vi "Actor Core.vi"(8 "error in":errorcluster, 11 "Nested in":refnum<class "Chef Actor.lvclass">) -> (0 "error out":errorcluster, 3 "Actor out":refnum<class "Actor.lvclass">)   [LabVIEW 2024, in "Chef Actor.lvlib" / "Chef Actor.lvclass"]
doc: "(<B>Filename</B>: Actor Framework.lvlib:Actor.lvclass:Actor Core.vi)\n\nReceives messages to the actor, reacts to them, and initiates any error handling that may shut the actor down.\n\nDescendant classes may override this VI to append parallel tasks for the actor to complete while it handles messages. Overrides use the Call Parent Method node."
uses:
  Chef Actor.lvclass
  C:/Program Files/National Instruments/LabVIEW 2024/vi.lib/ActorFramework/Actor/Actor.lvclass
  <vilib>/ActorFramework/Actor/Actor.lvclass
  Support/Step.ctl
  Timer/Timer/Timer.lvclass
  Cooker Actor/Cooker Actor.lvclass
  <vilib>/ActorFramework/Actor/Actor.lvclass/Actor.ctl
  <vilib>/ActorFramework/Message Enqueuer/Message Enqueuer.lvclass/Message Enqueuer.ctl
  Chef Actor.lvclass/Chef Actor.ctl
  <vilib>/ActorFramework/Message Enqueuer/Message Priority.ctl
  Chef Actor Messages/Start Cooker Msg/Start Cooker Msg.lvclass/Start Cooker Msg.ctl
  Chef Actor Messages/Start Timer Msg/Start Timer Msg.lvclass/Start Timer Msg.ctl
  <vilib>/ActorFramework/Message Enqueuer/Init from Existing Queue.vi
  <vilib>/ActorFramework/Message Enqueuer/Enqueue.vi
  Chef Actor Messages/Stop Timer Msg/Stop Timer Msg.lvclass
  C:/Program Files/National Instruments/LabVIEW 2024/vi.lib/ActorFramework/Message/Message.lvclass
  <vilib>/ActorFramework/Stop Msg/Stop Msg.lvclass
  Chef Actor Messages/Start Cooker Msg/Start Cooker Msg.lvclass
  Chef Actor Messages/Start Timer Msg/Start Timer Msg.lvclass
  <vilib>/ActorFramework/Message Priority Queue/Priority Enqueue.vi
  <vilib>/ActorFramework/Message Enqueuer/Message Enqueuer.lvclass
panel:
  out "Real Elapsed Time":u32
  out "Start Time":u32
  in  "StepsTable":string[][](table)
  out "StepsControl":T1[](array[typedef]) {"Duration" min=0.0 max=100.0 format="%.2f"; "Fire" min=0.0 max=100.0 format="%.2f %"}
  in  "Exit Button":bool
  out "Go Next Step":bool
  out "Current Index":i32
  out "Elapsed TÝme - Signal":bool
  in  "Start Button":bool
  out "Time Elapsed":dbl min=0.0 max=100.0 format="%.4f"
  # "STEPS"
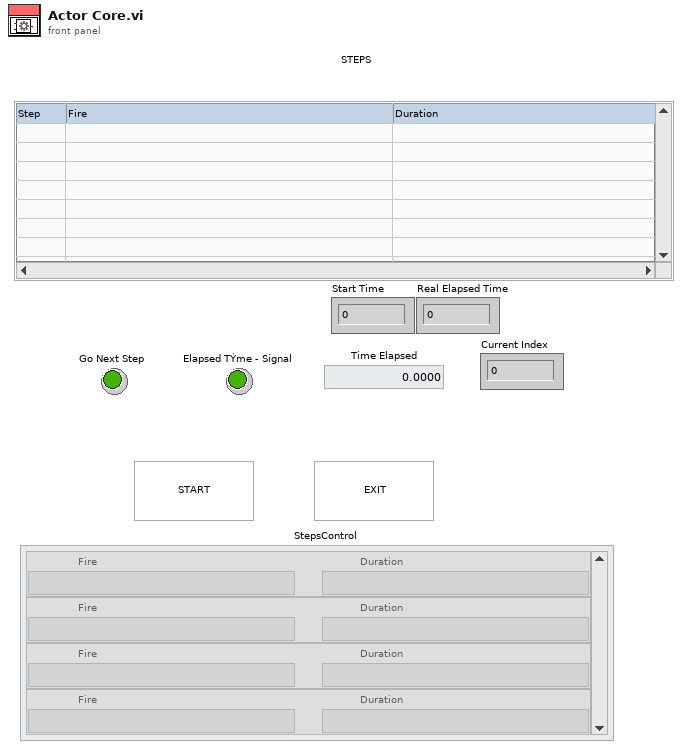
[diagram p1: front panel]
types:
  T1 = typedef "Step.ctl" = cluster{"Fire":dbl, "Duration":dbl}
  T2 = cluster{"Stop":refnum<user-event>, "Update Time Elapsed":refnum<user-event>, "Go Next Step":refnum<user-event>}
  T3 = typedef "Actor Framework.lvlib/Message Enqueuer.lvclass/Message Priority.ctl" = enum16{"Low", "Normal", "High"}
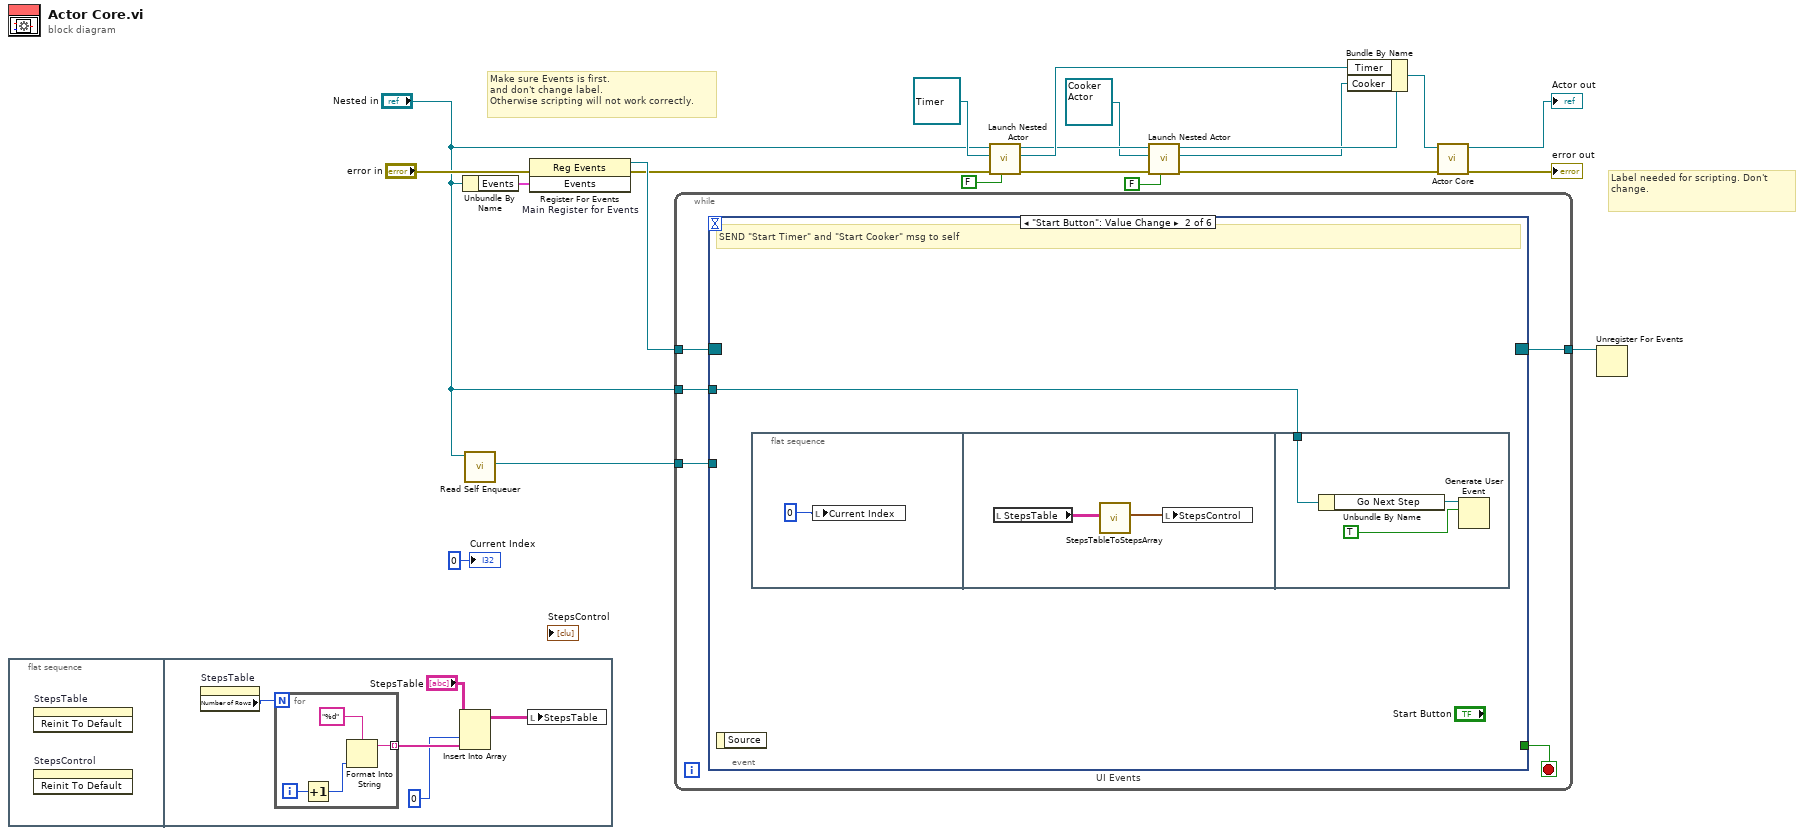
[diagram p0: block diagram]
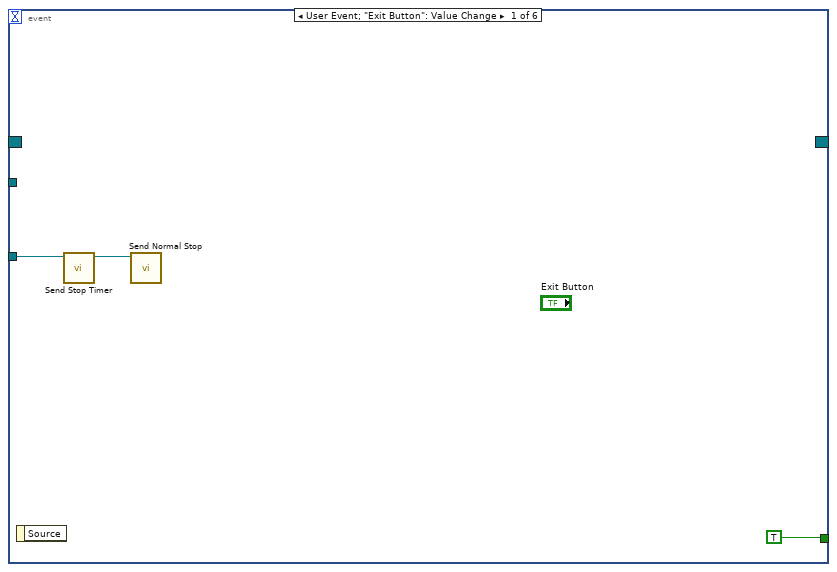
[diagram p2: hidden frame]
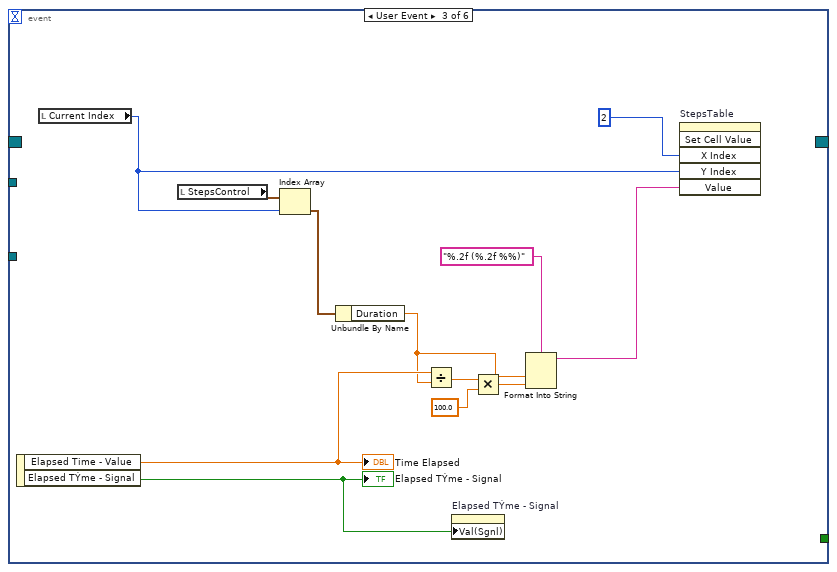
[diagram p3: hidden frame]
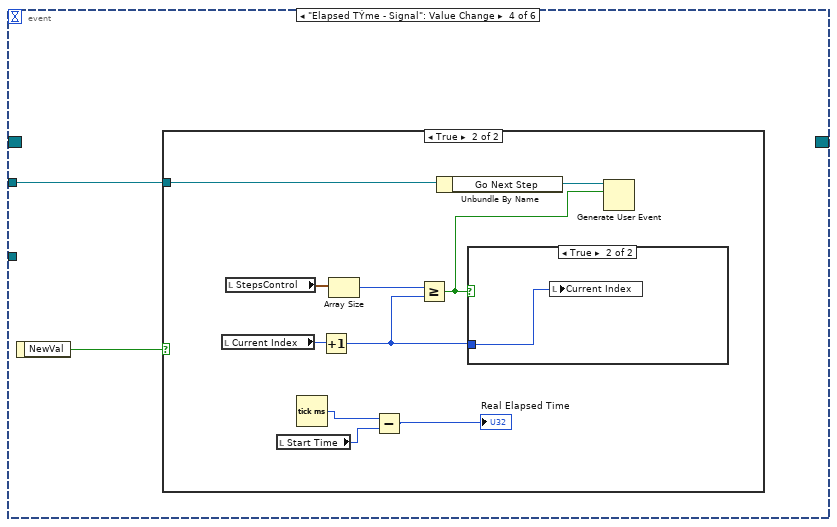
[diagram p4: hidden frame]
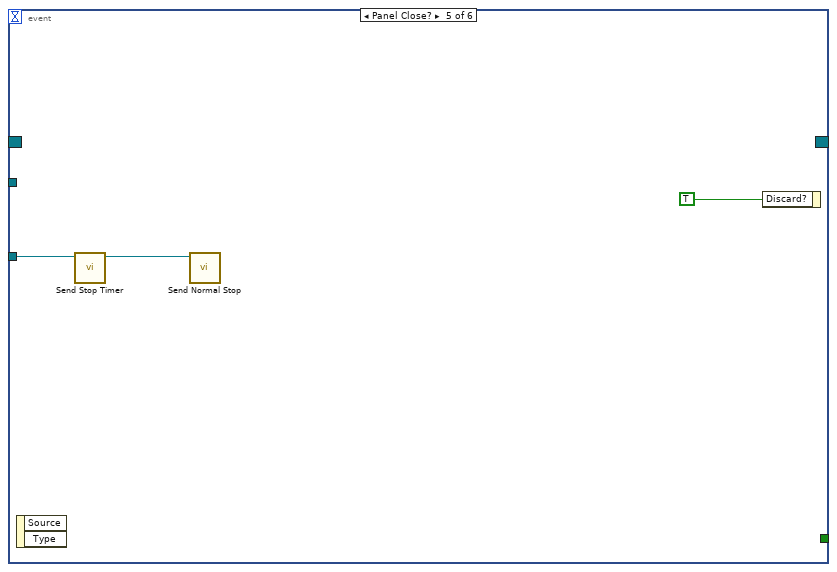
[diagram p7: hidden frame]
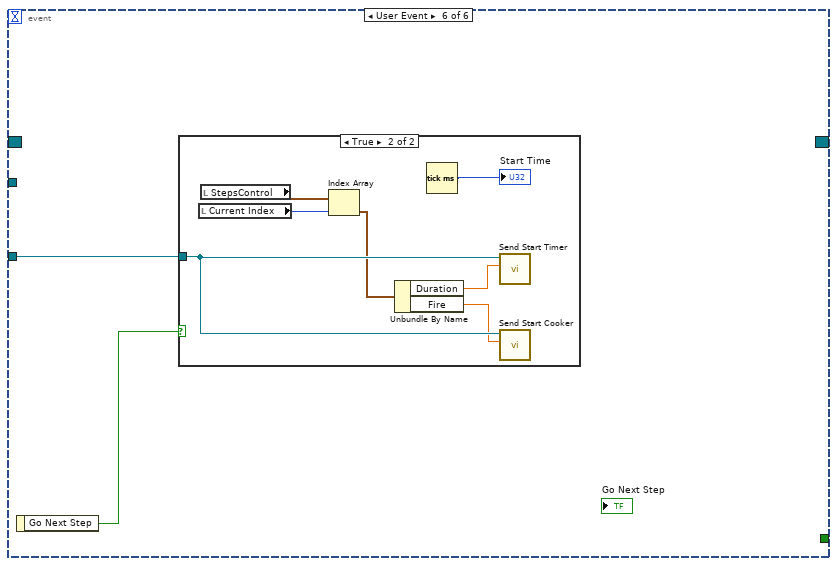
[diagram p8: hidden frame]
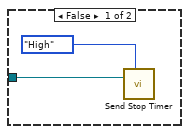
[diagram p9: hidden frame]
diagram:
  # "Label needed for scripting. Don't change."
  # "Make sure Events is first.\nand don't change label.\nOtherwise scripting will not work correctly."
  n1 = flat-sequence {
    frame #0 {
      n2 = invoke on="StepsTable" class="Tbl (strict)" method="Reinit To Default"() -> ()  [unwired: 3 in, 3 out]
      n3 = invoke on="StepsControl" class="Arr (strict)" method="Reinit To Default"() -> ()  [unwired: 3 in, 3 out]
    }
    frame #1 {
      n4 = property on="StepsTable" class="Tbl (strict)"() -> ("Number of Rows"=w22:u32)  [unwired: 2 in, 2 out]
      n5 = for {
        N: w22 -> [_]
        tunnel: [w28] -> w25 mode=indexing
        i -> [w30]
        n6 = Increment(x=w30) -> (x+1=w27:i32)
        n7 = Format Into String(format string="%d", w27) -> (resulting string=w28:string)  [unwired: 2 in, 1 out]
      }
      n8 = Insert Into Array(array="StepsTable", index (col)=0 ("index"), new element=w25) -> (w24:string[][])  [unwired: 1 in]
      n9 = local write "StepsTable"(w24) -> ()
    }
  }
  n10 = Unbundle By Name("Nested in") -> ("Events"=w18:T2)
  n11 = call <vilib>:"Read Self Enqueuer.vi"("Actor"="Nested in") -> ("Self Enqueuer"=w16:refnum<class "Message Enqueuer.lvclass">)  [unwired: 10 in]
  n12 = register-events "Main Register for Events"(error in="error in", w18) -> (reference out=w19:refnum<event-registration>, error out=w14:errorcluster)  [unwired: 1 in]
  n13 = while {
    tunnel: w19 -> [w35]
    tunnel: [w33] -> w17
    tunnel: w16 -> [w32]
    tunnel: "Nested in" -> [w31]
    stop <- w34 stop-if-true
    n14 = event "UI Events" shown="[1] \"Start Button\": Value Change" {
      selector: w35 -> [_ _ _ _ _ _]
      dyn-events: [_ _ _ _ _ _] -> w33
      timeout: _ -> [_ _ _ _ _ _]
      tunnel: [TRUE _ _ _ _ _] -> w34
      tunnel: w32 -> [w37 _ _ _ w72 w75]
      tunnel: w31 -> [_ w39 _ w59 _ _]
      event User Event; "Exit Button": Value Change {
        n15 = event-data() -> ()  [unwired: 1 in, 1 out]
        n16 = call "Send Stop Timer.vi"("Message Enqueuer"=w37) -> ("Message Enqueuer out"=w36:refnum<class "Message Enqueuer.lvclass">)  [unwired: 9 in, 1 out]
        n17 = call <vilib>:"Send Normal Stop.vi"("Message Enqueuer"=w36) -> ()  [unwired: 10 in, 1 out]
      }
      event "Start Button": Value Change {
        # "SEND \"Start Timer\" and \"Start Cooker\" msg to self"
        n18 = event-data() -> ()  [unwired: 1 in, 1 out]
        n19 = flat-sequence {
          tunnel: w39 -> [w45]
          frame #0 {
            n20 = local write "Current Index"(0 ("Current Index")) -> ()
          }
          frame #1 {
            n21 = local read "StepsTable"() -> (w42:string[][])
            n22 = call "StepsTableToStepsArray.vi"("Steps Table Input"=w42) -> ("Steps Array Output"=w41:T1[])  [unwired: 4 in]
            n23 = local write "StepsControl"(w41) -> ()
          }
          frame #2 {
            n24 = Unbundle By Name(w45) -> ("Go Next Step"=w44:refnum<user-event>)
            n25 = Generate User Event(user event=w44, event data cluster=TRUE ("event data")) -> ()  [unwired: 2 in, 2 out]
          }
        }
      }
      event User Event {
        n26 = event-data() -> ("Elapsed Time - Value"=w54:dbl, "Elapsed TÝme - Signal"=w57:bool)  [unwired: 1 in]
        "Time Elapsed" <- w54
        "Elapsed TÝme - Signal" <- w57
        n27 = local read "Current Index"() -> (w46:i32)
        n28 = local read "StepsControl"() -> (w56:T1[])
        n29 = Index Array(array=w56, index=w46) -> (element=w55:T1)
        n30 = Unbundle By Name(w55) -> ("Duration"=w49:dbl)
        n31 = Divide(x=w54, y=w49) -> (x/y=w53:dbl)
        n32 = property on="Elapsed TÝme - Signal" class="Bool (strict)"("Val(Sgnl)"=w57) -> ()  [unwired: 2 in, 2 out]
        n33 = Multiply(x=w53, y=100.0) -> (x*y=w50:dbl)
        n34 = Format Into String(format string="%.2f (%.2f %%)", w49, w50) -> (resulting string=w48:string)  [unwired: 2 in, 1 out]
        n35 = invoke on="StepsTable" class="Tbl (strict)" method="Set Cell Value"("X Index"=2 ("index (col)"), "Y Index"=w46, "Value"=w48) -> ()  [unwired: 3 in, 6 out]
      }
      event "Elapsed TÝme - Signal": Value Change {
        n36 = event-data() -> ("NewVal"=w58:bool)  [unwired: 1 in]
        n37 = case shown="True" w58 {
          tunnel: w59 -> [_ w65]
          frame False {
          }
          frame True {
            n38 = local read "Current Index"() -> (w69:i32)
            n39 = local read "StepsControl"() -> (w67:T1[])
            n40 = local read "Start Time"() -> (w62:u32)
            n41 = Tick Count (ms)() -> (millisecond timer value=w61:u32)
            n42 = Increment(x=w69) -> (x+1=w64:i32)
            n43 = Array Size(array=w67) -> (size(s)=w66:i32)
            n44 = Subtract(x=w61, y=w62) -> (x-y=→"Real Elapsed Time":u32)
            n45 = Greater Or Equal?(x=w66, y=w64) -> (x >= y?=w63:bool)
            n46 = Unbundle By Name(w65) -> ("Go Next Step"=w68:refnum<user-event>)
            n47 = case shown="True" w63 {
              tunnel: w64 -> [_ w70]
              frame False {
              }
              frame True {
                n48 = local write "Current Index"(w70) -> ()
              }
            }
            n49 = Generate User Event(user event=w68, event data cluster=w63) -> ()  [unwired: 2 in, 2 out]
          }
        }
      }
      event Panel Close? {
        n50 = event-data() -> ()  [unwired: 1 in, 2 out]
        n51 = call "Send Stop Timer.vi"("Message Enqueuer"=w72) -> ("Message Enqueuer out"=w71:refnum<class "Message Enqueuer.lvclass">)  [unwired: 9 in, 1 out]
        n52 = call <vilib>:"Send Normal Stop.vi"("Message Enqueuer"=w71) -> ()  [unwired: 10 in, 1 out]
        n53 = event-data("Discard?"=TRUE) -> ()  [unwired: 1 in, 1 out]
      }
      event User Event {
        n54 = event-data() -> ("Go Next Step"=w74:bool)  [unwired: 1 in]
        n55 = case shown="True" w74 {
          tunnel: w75 -> [w77 w84]
          frame False {
            n56 = call "Send Stop Timer.vi"("Message Priority (Normal)"=Message_Priority."High", "Message Enqueuer"=w77) -> ()  [unwired: 8 in, 2 out]
          }
          frame True {
            n57 = local read "Current Index"() -> (w83:i32)
            n58 = local read "StepsControl"() -> (w82:T1[])
            n59 = Index Array(array=w82, index=w83) -> (element=w81:T1)
            n60 = Unbundle By Name(w81) -> ("Duration"=w80:dbl, "Fire"=w79:dbl)
            n61 = Tick Count (ms)() -> (millisecond timer value=→"Start Time":u32)
            n62 = call "Send Start Timer.vi"("Duration"=w80, "Message Enqueuer"=w84) -> ()  [unwired: 8 in, 2 out]
            n63 = call "Send Start Cooker.vi"("Fire"=w79, "Message Enqueuer"=w84) -> ()  [unwired: 8 in, 2 out]
          }
        }
      }
    }
  }
  n64 = call <vilib>:"Launch Nested Actor.vi"("Open Actor Core front panel? (F)"=FALSE, "error in (no error)"=w14, "Nested Actor"=refnum<class "Timer.lvclass"> refnum ("Timer.lvlib:Timer.lvclass"), "Caller Actor in"="Nested in") -> ("error out"=w10:errorcluster, "Nested Actor's Enqueuer"=w11:refnum<class "Message Enqueuer.lvclass">, "Caller Actor out"=w9:refnum<class "Chef Actor.lvclass">)  [unwired: 5 in]
  n65 = call <vilib>:"Launch Nested Actor.vi"("Open Actor Core front panel? (F)"=FALSE, "error in (no error)"=w10, "Nested Actor"=refnum<class "Cooker Actor.lvclass"> refnum ("Cooker Actor.lvlib:Cooker Actor.lvclass"), "Caller Actor in"=w9) -> ("error out"=w7:errorcluster, "Nested Actor's Enqueuer"=w5:refnum<class "Message Enqueuer.lvclass">, "Caller Actor out"=w8:refnum<class "Chef Actor.lvclass">)  [unwired: 5 in]
  n66 = Bundle By Name(cluster=w8, "Timer"=w11, "Cooker"=w5) -> (w12:refnum<class "Chef Actor.lvclass">)
  n67 = call-parent "Actor Core.vi"("error in"=w7, "Actor in"=w12) -> ("error out"=→"error out":errorcluster, "Actor out"=→"Actor out":refnum<class "Actor.lvclass">)  [unwired: 8 in]
  n68 = Unregister For Events(event registration refnum=w17) -> ()  [unwired: 1 in, 1 out]
  "Current Index" <- 0 ("Current Index")
